vi "Report_Font_wizard.vi"(2 "error in (no error)":errorcluster, 4 "font in":T1={"font name"="", "font size"=0.0, "bold"=0, "italic"=0, "underline"=0, "strike through"=0, "font color"=16777216} caption="font" {"font size" format="%0.2f"; "strike through" items=["Unchanged", "Yes", "No"]; "underline" items=["Unchanged", "Yes", "No"]; "italic" items=["Unchanged", "Yes", "No"]; "bold" items=["Unchanged", "Yes", "No"]}) -> (0 "error out":errorcluster, 1 "font out":T1={"font name"="", "font size"=0.0, "bold"=0, "italic"=0, "underline"=0, "strike through"=0, "font color"=16777216} caption="font" {"font size" format="%0.2f"; "strike through" items=["Unchanged", "Yes", "No"]; "underline" items=["Unchanged", "Yes", "No"]; "italic" items=["Unchanged", "Yes", "No"]; "bold" items=["Unchanged", "Yes", "No"]})   [LabVIEW 2020, in "NI_ReportGenerationToolkit.lvlib"]
uses:
  <vilib>/addons/_office/NI_ReportGenerationToolkit.lvlib
  <vilib>/addons/_office/_exclsub.llb/font.ctl
panel:
  in  "MSComDlg.ICommonDialog":refnum<k7>
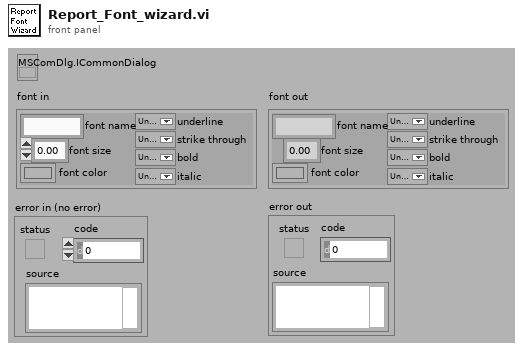
[diagram p1: front panel]
types:
  T1 = typedef "NI_ReportGenerationToolkit.lvlib/font.ctl" = cluster{"font name":string, "font size":dbl, "bold":u16, "italic":u16, "underline":u16, "strike through":u16, "font color":u32}
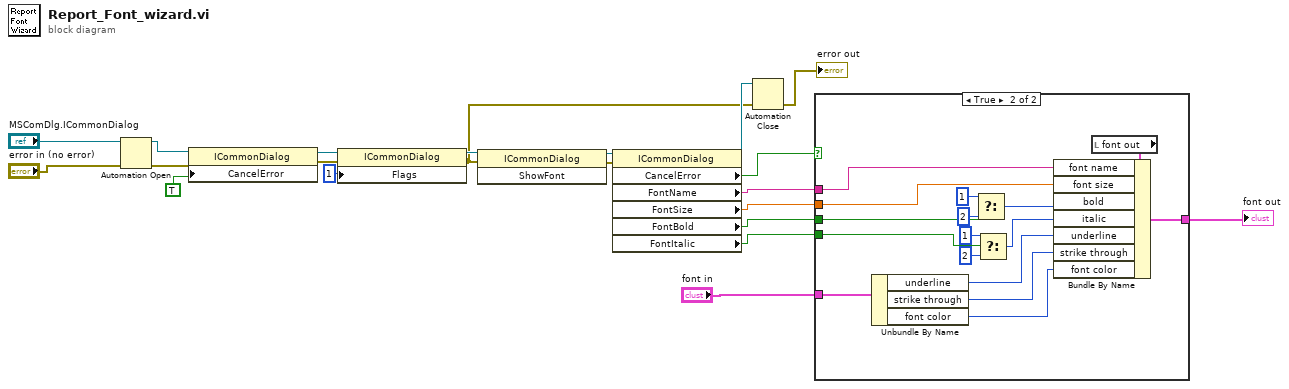
[diagram p0: block diagram]
diagram:
  n1 = Automation Open(error in (no error)="error in (no error)", Automation Refnum="MSComDlg.ICommonDialog") -> (Automation Refnum=w20:refnum<k7>, error out=w19:errorcluster)  [unwired: 2 in]
  n2 = property class="ICommonDialog"(reference=w20, error in=w19, "CancelError"=TRUE) -> (reference out=w17:refnum<k7>, error out=w16:errorcluster)
  n3 = property class="ICommonDialog"(reference=w17, error in=w16, "Flags"=1) -> (reference out=w15:refnum<k7>, error out=w2:errorcluster)
  n4 = invoke class="ICommonDialog" method="ShowFont"(reference=w15, error in=w2) -> (reference out=w8:refnum<k7>, error out=w3:errorcluster)  [unwired: 1 in, 1 out]
  n5 = property class="ICommonDialog"(reference=w8, error in=w3) -> (reference out=w6:refnum<k7>, "CancelError"=w4:bool, "FontName"=w7:string, "FontSize"=w12:sgl, "FontBold"=w11:bool, "FontItalic"=w10:bool)  [unwired: 1 out]
  n6 = Automation Close(3:w2, 5:w6) -> (0:→"error out":errorcluster)
  n7 = case shown="True" w4 {
    tunnel: w12 -> [_ w37]
    tunnel: w11 -> [_ w36]
    tunnel: w10 -> [_ w32]
    tunnel: [w22 w28] -> w9
    tunnel: w7 -> [_ w27]
    tunnel: "font in" -> [w22 w26]
    frame False {
    }
    frame True {
      n8 = Unbundle By Name(w26) -> ("underline"=w25:u16, "strike through"=w24:u16, "font color"=w23:u32)
      n9 = Select(t=1, s=w36, f=2 ("t")) -> (s? t:f=w33:i32)
      n10 = Select(t=1, s=w32, f=2 ("t")) -> (s? t:f=w30:i32)
      n11 = local read "font out"() -> (w38:T1)
      n12 = Bundle By Name(cluster=w38, "font name"=w27, "font size"=w37, "bold"=w33, "italic"=w30, "underline"=w25, "strike through"=w24, "font color"=w23) -> (w28:T1)
    }
  }
  "font out" <- w9
